vi "HexFile.vi"(5 "Offset":cluster{"Angle":sgl, "AngEle":sgl, "RCS":sgl}[](array[cluster]), 6 "Data Log Path":path, 7 "SN":string, 8 "error in (no error)":errorcluster, 9 "Boolean":bool, 10 "RFPayloads":u8[](array[numeric]) format="%.0x", 11 "calibration_parameters":T1[](array[typedef])=[{"re"=1.0, "im"=0.0}, {"re"=-0.96036863, "im"=0.2425586}, {"re"=0.9626107, "im"=-0.2713669}, {"re"=-0.58503306, "im"=0.7473227}, {"re"=1.0340631, "im"=-0.051051468}, {"re"=-0.9827397, "im"=0.29056582}, {"re"=0.9798006, "im"=-0.31922665}, {"re"=-0.5774226, "im"=0.79138196}, {"re"=0.83439076, "im"=0.47953746}, {"re"=-0.9034144, "im"=-0.2641089}, {"re"=0.9161487, "im"=0.24367115}, {"re"=-0.8432455, "im"=0.32213277}, {"re"=0.39170918, "im"=0.81630135}, {"re"=-0.566318, "im"=-0.6832286}, {"re"=0.58235455, "im"=0.6756262}, {"re"=-0.82617307, "im"=-0.19347626}]) -> (0 "error out":errorcluster, 3 "hex file path":path)   [LabVIEW 2024]
uses:
  Controls/Calc Para_float.ctl
panel:
  out "calibration_parameters_radar":i32[](array[numeric])
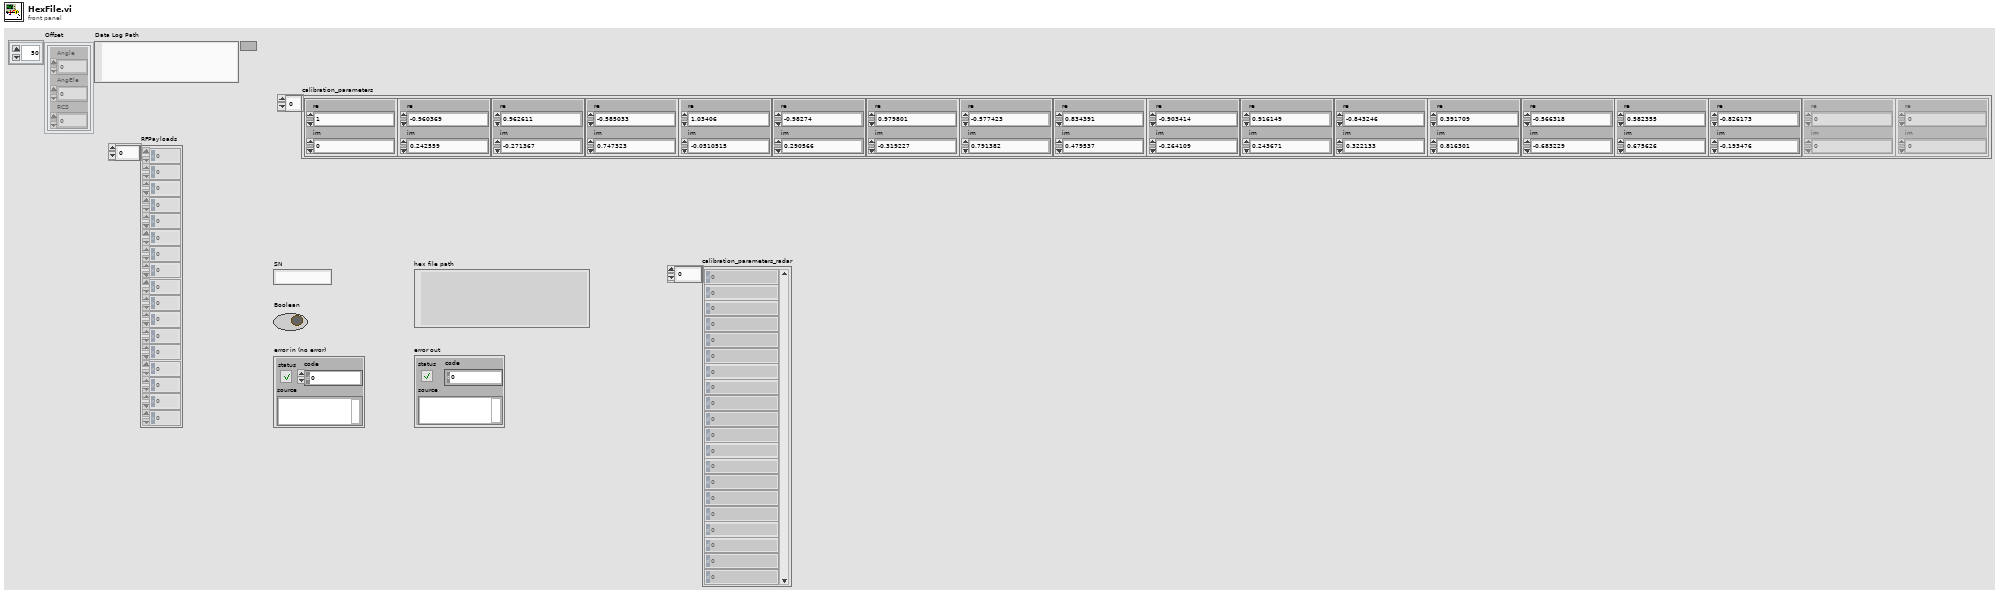
[diagram p1: front panel]
types:
  T1 = typedef "Calc Para_float.ctl" = cluster{"re":sgl, "im":sgl}
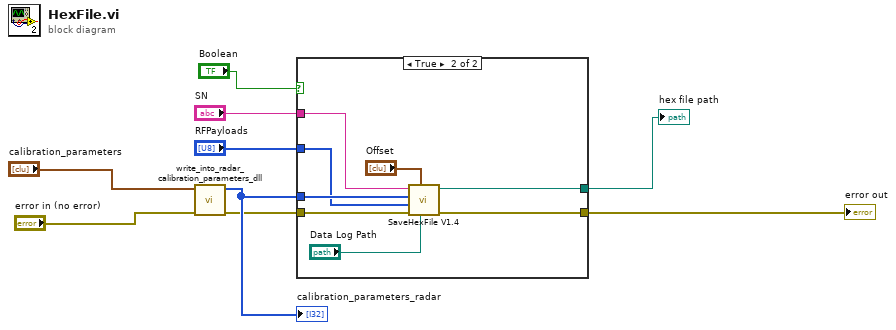
[diagram p0: block diagram]
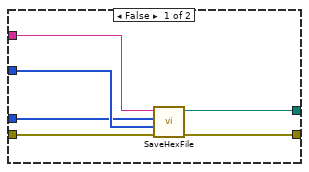
[diagram p2: hidden frame]
diagram:
  n1 = call "write_into_radar_calibration_parameters_dll.vi"("error in (no error)"="error in (no error)", "calibration_parameters"="calibration_parameters") -> ("error out"=w7:errorcluster, "calibration_parameters_radar"=w8:i32[])  [unwired: 7 in, 1 out]
  "calibration_parameters_radar" <- w8
  n2 = case shown="True" "Boolean" {
    tunnel: w8 -> [w10 w23]
    tunnel: w7 -> [w15 w22]
    tunnel: [w14 w21] -> w6
    tunnel: "SN" -> [w12 w20]
    tunnel: "RFPayloads" -> [w11 w19]
    tunnel: [w13 w18] -> w2
    frame False {
      n3 = call "SaveHexFile.vi"("error IO"=w15, "RFPayloads"=w11, "calibration_parameters_radar"=w10, "SN"=w12) -> ("error out"=w14:errorcluster, "hex file path"=w13:path)  [unwired: 6 in]
    }
    frame True {
      n4 = call "SaveHexFile V1.4.vi"("Data Log Path"="Data Log Path", "Offset"="Offset", "error IO"=w22, "RFPayloads"=w19, "calibration_parameters_radar"=w23, "SN"=w20) -> ("error out"=w21:errorcluster, "hex file path"=w18:path)  [unwired: 4 in]
    }
  }
  "error out" <- w6
  "hex file path" <- w2
